vi "reset DRV UI (SubVI).vi"(11 "Ref  in":refnum<vi>[](array[refnum])) -> (0 "error out":errorcluster, 3 "Ref out":refnum<vi>[](array[refnum]))   [LabVIEW 2018, in "Application.lvlib"]
uses:
  Application.lvlib
panel:
  in  "error in (no error)":errorcluster
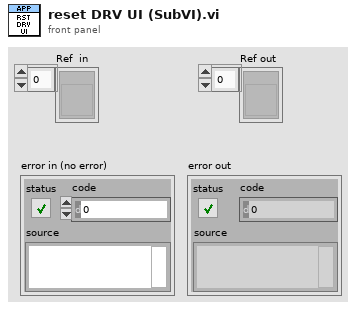
[diagram p1: front panel]
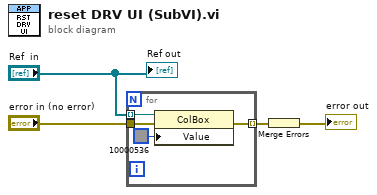
[diagram p0: block diagram]
diagram:
  n1 = for {
    tunnel: "Ref  in" -> [w7] mode=indexing
    tunnel: [w6] -> w3 mode=indexing
    tunnel: "error in (no error)" -> [w5]
    n2 = property class="ColBox"(reference=w7, error in=w5, "Value"=u32 10000536 ("DRV 1")) -> (error out=w6:errorcluster)  [unwired: 1 out]
  }
  n3 = Merge Errors(w3) -> (→"error out":errorcluster)
  "Ref out" <- "Ref  in"
